vi "Get Variables.vi"(8 "error in (no error)":errorcluster, 11 "Comparison Operations in":refnum<class "Comparison Operations.lvclass">) -> (0 "error out":errorcluster, 2 "Variables":variant, 3 "Comparison Operations out":refnum<class "Comparison Operations.lvclass">)   [LabVIEW 2016, in "Comparison Operations.lvclass"]
uses:
  Comparison Operations.lvclass
  Comparison Operations.lvclass/Comparison Operations.ctl
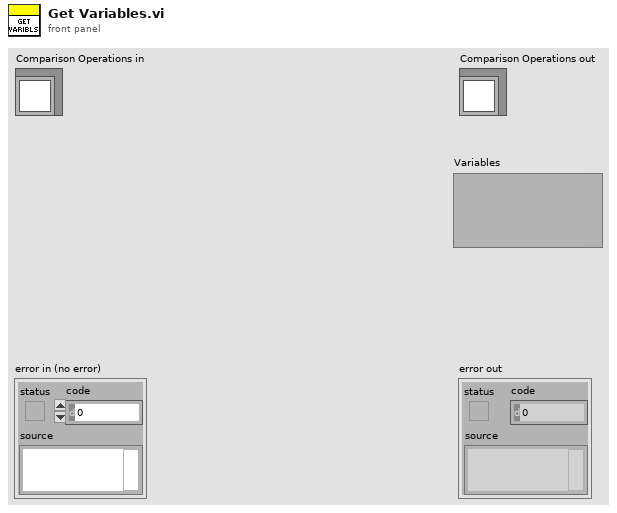
[diagram p1: front panel]
types:
  T1 = typedef "Comparison Operations.lvclass/Variables.ctl" = cluster{"Var1":variant, "Var2":variant}
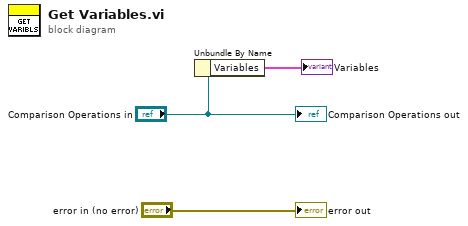
[diagram p0: block diagram]
diagram:
  n1 = Unbundle By Name("Comparison Operations in") -> ("Variables"=→"Variables":T1)
  "error out" <- "error in (no error)"
  "Comparison Operations out" <- "Comparison Operations in"
